vi "Initialise Front Panel.vi"(7 "This VI":refnum<vi>, 11 "UI Ref":T1) -> (0 "error out":errorcluster)   [LabVIEW 2021]
uses:
  Controls/UI References.ctl
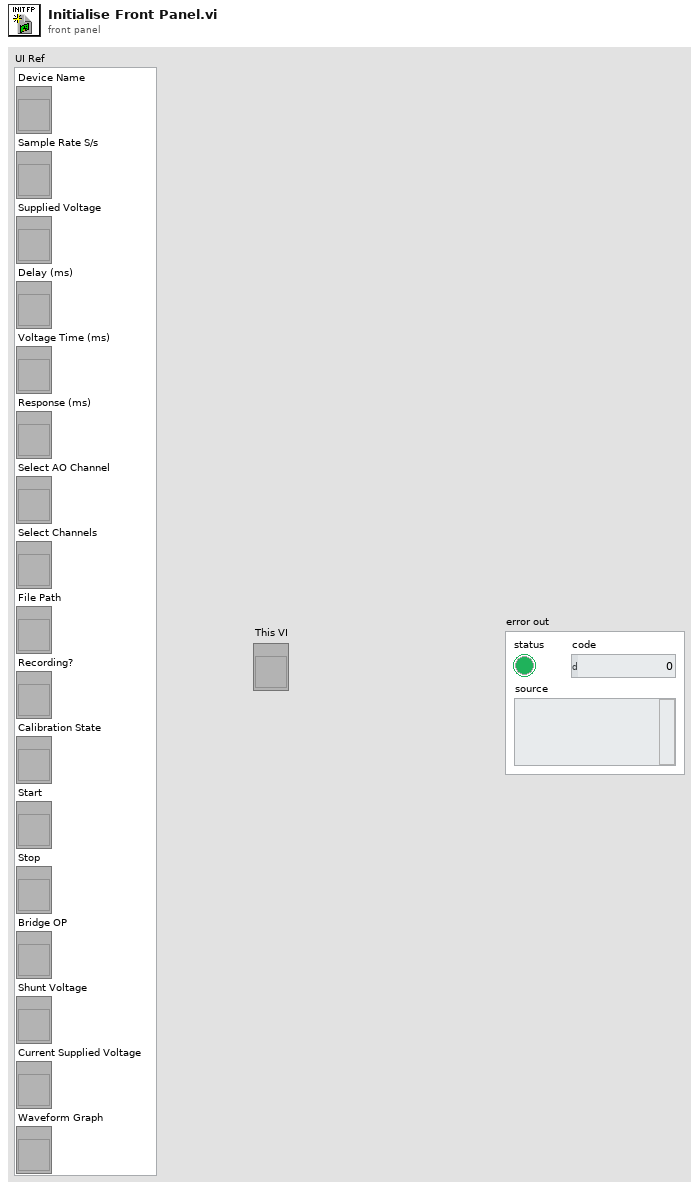
[diagram p1: front panel]
types:
  T1 = typedef "UI References.ctl" = cluster{"Device Name":refnum<vi>, "Sample Rate S/s":refnum<vi>, "Supplied Voltage":refnum<vi>, "Delay (ms)":refnum<vi>, "Voltage Time (ms)":refnum<vi>, "Response (ms)":refnum<vi>, "Select AO Channel":refnum<vi>, "Select Channels":refnum<vi>, "File Path":refnum<vi>, "Recording?":refnum<vi>, "Calibration State":refnum<vi>, "Start":refnum<vi>, "Stop":refnum<vi>, "Bridge OP":refnum<vi>, "Shunt Voltage":refnum<vi>, "Current Supplied Voltage ":refnum<vi>, "Waveform Graph":refnum<vi>}
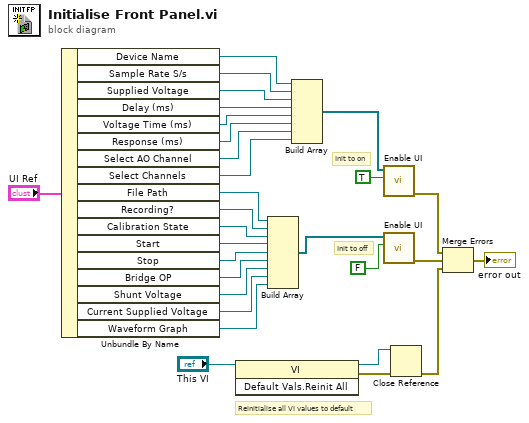
[diagram p0: block diagram]
diagram:
  # "Init to on"
  # "Init to off"
  # "Reinitialise all VI values to default"
  n1 = Unbundle By Name("UI Ref") -> ("Device Name"=w19:refnum<vi>, "Sample Rate S/s"=w18:refnum<vi>, "Supplied Voltage"=w17:refnum<vi>, "Delay (ms)"=w16:refnum<vi>, "Voltage Time (ms)"=w15:refnum<vi>, "Response (ms)"=w14:refnum<vi>, "Select AO Channel"=w13:refnum<vi>, "Select Channels"=w12:refnum<vi>, "File Path"=w11:refnum<vi>, "Recording?"=w10:refnum<vi>, "Calibration State"=w9:refnum<vi>, "Start"=w8:refnum<vi>, "Stop"=w7:refnum<vi>, "Bridge OP"=w6:refnum<vi>, "Shunt Voltage"=w5:refnum<vi>, "Current Supplied Voltage"=w4:refnum<vi>, "Waveform Graph"=w3:refnum<vi>)
  n2 = invoke class="VI" method="Default Vals.Reinit All"(reference="This VI") -> (reference out=w28:refnum<vi>, error out=w25:errorcluster)  [unwired: 2 in, 1 out]
  n3 = Build Array(w11, w10, w9, w8, w7, w6, w5, w4, w3) -> (w1:refnum<vi>[])
  n4 = Build Array(w19, w18, w17, w16, w15, w14, w13, w12) -> (w2:refnum<vi>[])
  n5 = call "Enable UI.vi"("Enable?"=TRUE, "output cluster"=w2) -> ("error out"=w24:errorcluster)  [unwired: 9 in]
  n6 = call "Enable UI.vi"("Enable?"=FALSE, "output cluster"=w1) -> ("error out"=w23:errorcluster)  [unwired: 9 in]
  n7 = Close Reference(reference=w28, error in (no error)=w25) -> (error out=w22:errorcluster)
  n8 = Merge Errors(w24, w23, w22) -> (→"error out":errorcluster)
